vi "Set - SigMath Data.vi"(0 "reference in":refnum<class "SigMath.lvclass">, 5 "error in (no error)":errorcluster, 7 "SigMath Data":T1) -> (14 "reference out":refnum<class "SigMath.lvclass">, 19 "error out":errorcluster)   [LabVIEW 2022 SP3, in "SigMath.lvclass"]
uses:
  SigMath.lvclass
  protected/SigMath Data.ctl
  API/GSwFormDSP_class/GSwFormDSP.lvclass
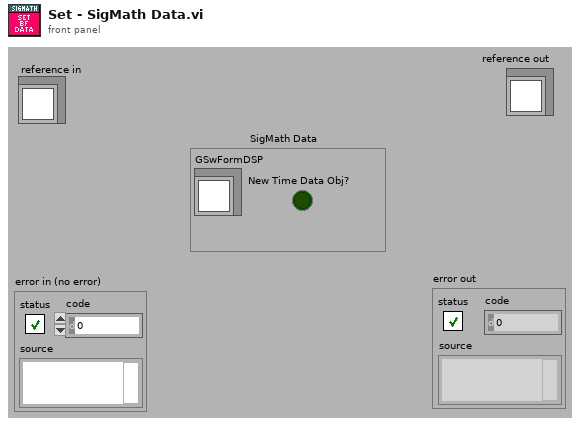
[diagram p1: front panel]
types:
  T1 = typedef "SigMath.lvclass/SigMath Data.ctl" = cluster{"New Time Data Obj?":bool, "GSwFormDSP":refnum<class "GSwFormDSP.lvclass">}
  T2 = typedef "SigMath.lvclass/ObjectAttributesRef.ctl" = refnum<data-value>
  T3 = typedef "SigMath.lvclass/ObjectAttributes.ctl" = cluster{"SigMath Data":T1, "User CTRL Refs":T4}
  T4 = typedef "SigMath.lvclass/SigMath User CTRL Refs.ctl" = cluster{"wForms":refnum<vi>, "Results wForms":refnum<vi>}
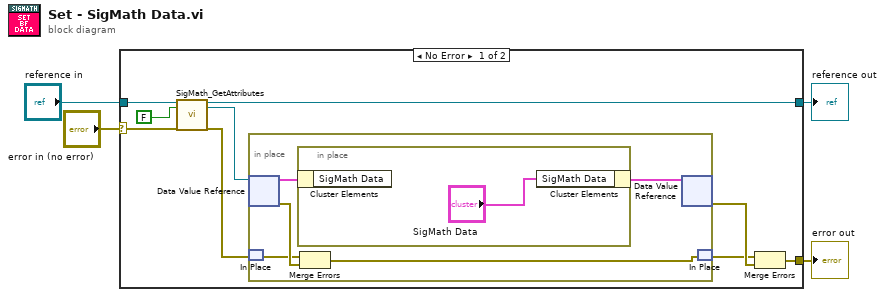
[diagram p0: block diagram]
diagram:
  n1 = case shown="No Error" "error in (no error)" {
    selector: "error in (no error)" -> [w9 w21]
    tunnel: [w13 w21] -> w3
    tunnel: [w8 w20] -> w1
    tunnel: "reference in" -> [w11 w20]
    frame No Error {
      n2 = call "SigMath_GetAttributes.vi"("reference in"=w11, "return data? (T)"=FALSE, "error in (no error)"=w9) -> ("reference out"=w8:refnum<class "SigMath.lvclass">, "attributes ref"=w7:T2, "error out"=w6:errorcluster)  [unwired: 13 in, 1 out]
      n3 = in-place {
        n4 = in-place-dvr #1(w7) -> (w17:T3, w16:errorcluster)
        n5 = in-place-match #2(w6) -> (w15:errorcluster)
        n6 = in-place {
          n7 = in-place-cluster #3(w17) -> ()  [unwired: 1 out]
          n8 = in-place-cluster #3("SigMath Data"="SigMath Data") -> (w18:T3)
        }
        n9 = Merge Errors(w15, w16) -> (w14:errorcluster)
        n10 = in-place-dvr #1(w18) -> (w12:errorcluster)  [unwired: 1 out]
        n11 = in-place-match #2(w14) -> (w5:errorcluster)
      }
      n12 = Merge Errors(w5, w12) -> (w13:errorcluster)
    }
    frame Error {
    }
  }
  "error out" <- w3
  "reference out" <- w1
